vi "Rx.vi"(0 "rx.parameters":T6={"rx.trigger select"=enum."Software", "rx.trigger enable"=FALSE, "rx.trigger sync enable"=FALSE, "rx 0.stream enable"=FALSE, "rx 1.stream enable"=FALSE, "rx.software trigger"=FALSE, "rx.reset"=FALSE, "rx.abort"=FALSE, "rx.samples to acquire"=0, "ddc parameters"=[{"output sample rate"=0.0, "delay"=0.0, "frequency shift"=0.0, "impairments"={"inline gain I"=0.0, "inline gain Q"=0.0, "cross gain I"=0.0, "cross gain Q"=0.0, "pre-gain offset I"=0.0, "pre-gain offset Q"=0.0, "post-gain offset I"=0.0, "post-gain offset Q"=0.0}, "phase"=0.0}, {"output sample rate"=0.0, "delay"=0.0, "frequency shift"=0.0, "impairments"={"inline gain I"=0.0, "inline gain Q"=0.0, "cross gain I"=0.0, "cross gain Q"=0.0, "pre-gain offset I"=0.0, "pre-gain offset Q"=0.0, "post-gain offset I"=0.0, "post-gain offset Q"=0.0}, "phase"=0.0}]} {"ddc parameters"."frequency shift" format="%#.48g"}, 5 "rx.start trigger":bool) -> (4 "rx.status":T2)   [LabVIEW 2023]
uses:
  <instrlib>/_niInstr/DSP/v1/Shared/Public/IQ Impairments.ctl
  <instrlib>/niUSRP/Reference FPGA/USRPRIO Sample VIs/FPGA/SubVIs/DDC Parameters.ctl
  <instrlib>/niUSRP/Reference FPGA/USRPRIO Sample VIs/Host/SubVIs/Start Trigger.ctl
  <instrlib>/niUSRP/Reference FPGA/USRPRIO Sample VIs/FPGA/SubVIs/Stream Control State.ctl
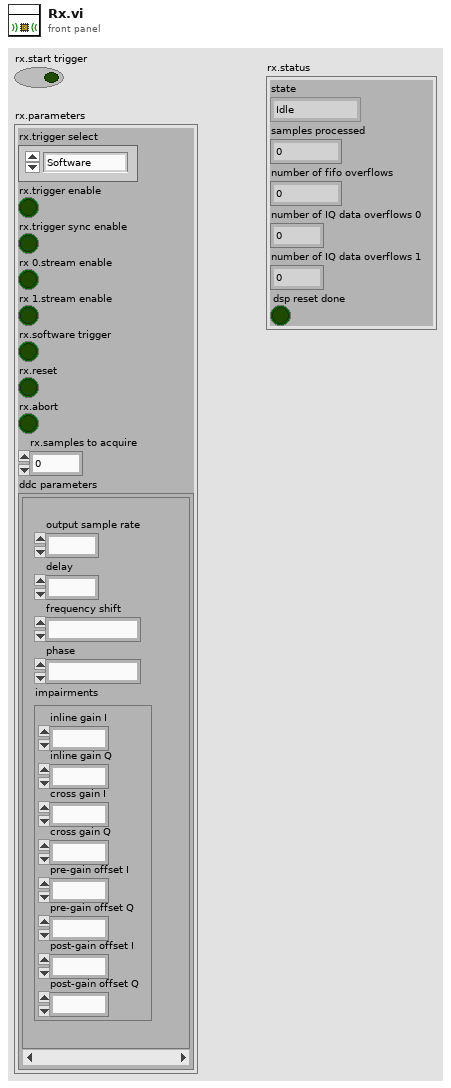
[diagram p1: front panel]
types:
  T1 = typedef "Stream Control State.ctl" = enum16{"Idle", "Active"}
  T2 = cluster{"state":T1, "samples processed":u32, "number of fifo overflows":u32, "number of IQ data overflows 0":u64, "number of IQ data overflows 1":u64, "dsp reset done":bool}
  T3 = typedef "Start Trigger.ctl" = enum8{"Software", "Digital Edge", "Rx Start Trigger", "Tx Start Trigger", "Immediate", "Future Time Event"}
  T4 = typedef "DDC Parameters.ctl" = cluster{"output sample rate":fxp<+,48,1>, "delay":fxp<+/-,16,0>, "frequency shift":fxp<+/-,48,0>, "impairments":T5, "phase":fxp<+/-,21,0>}
  T5 = typedef "niInstr DSP v1 Shared.lvlib/IQ Impairments.ctl" = cluster{"inline gain I":fxp<+/-,18,1>, "inline gain Q":fxp<+/-,18,1>, "cross gain I":fxp<+/-,18,1>, "cross gain Q":fxp<+/-,18,1>, "pre-gain offset I":fxp<+/-,18,1>, "pre-gain offset Q":fxp<+/-,18,1>, "post-gain offset I":fxp<+/-,18,1>, "post-gain offset Q":fxp<+/-,18,1>}
  T6 = cluster{"rx.trigger select":T3, "rx.trigger enable":bool, "rx.trigger sync enable":bool, "rx 0.stream enable":bool, "rx 1.stream enable":bool, "rx.software trigger":bool, "rx.reset":bool, "rx.abort":bool, "rx.samples to acquire":u32, "ddc parameters":T4[]}
  T7 = cluster{"rx.state":T1, "rx.samples processed":u32, "rx.number of fifo overflows":u32, "rx 0.number of IQ data overflows":u64, "rx 1.number of IQ data overflows":u64, "rx.dsp reset done":bool}
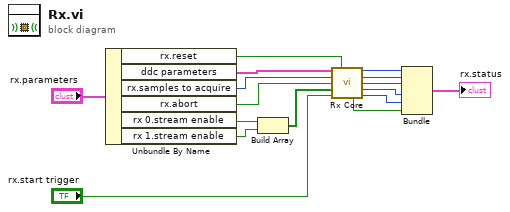
[diagram p0: block diagram]
diagram:
  n1 = Unbundle By Name("rx.parameters") -> ("rx.reset"=w12:bool, "ddc parameters"=w15:T4[], "rx.samples to acquire"=w14:u32, "rx.abort"=w13:bool, "rx 0.stream enable"=w11:bool, "rx 1.stream enable"=w10:bool)
  n2 = Build Array(w11, w10) -> (w9:bool[])
  n3 = call <instrlib>:"Rx Core.vi"("ddc parameters"=w15, "rx.reset"=w12, "rx.samples to acquire"=w14, "rx.abort"=w13, "rx.stream enable"=w9, "rx.start trigger"="rx.start trigger") -> ("rx.state"=w7:T1, "rx.samples processed"=w6:u32, "rx.number of fifo overflows"=w5:u32, "rx 0.number of IQ data overflows"=w4:u64, "rx.dsp reset done"=w2:bool, "rx 1.number of IQ data overflows"=w3:u64)  [unwired: 4 in]
  n4 = Bundle("rx.state"=w7, "rx.samples processed"=w6, "rx.number of fifo overflows"=w5, "rx 0.number of IQ data overflows"=w4, "rx 1.number of IQ data overflows"=w3, "rx.dsp reset done"=w2) -> (→"rx.status":T7)  [unwired: 1 in]
